vi "buildWaveform.vi"(8 "error in (no error)":errorcluster, 10 "Waveforms":T1, 11 "WaveformFactory in":refnum<class "WaveformFactory.lvclass">) -> (0 "error out":errorcluster, 2 "Waveform":refnum<class "IWaveform.lvclass">, 3 "WaveformFactory out":refnum<class "WaveformFactory.lvclass">)   [LabVIEW 2015, in "WaveformFactory.lvclass"]
uses:
  WaveformFactory.lvclass
  Typedefs/Waveform.ctl
  Waveforms/IWaveforms/IWaveform.lvclass
  WaveformFactory.lvclass/WaveformFactory.ctl
  Waveforms/PeriodicWave/PeriodicWave.lvclass
  Waveforms/ChirpWave/ChirpWave.lvclass
  Waveforms/GuassianNoiseWave/GuassianNoiseWave.lvclass
  Waveforms/TrapezoidalWave/TrapezoidalWave.lvclass
  Typedefs/FAMTTypedefs.lvlib
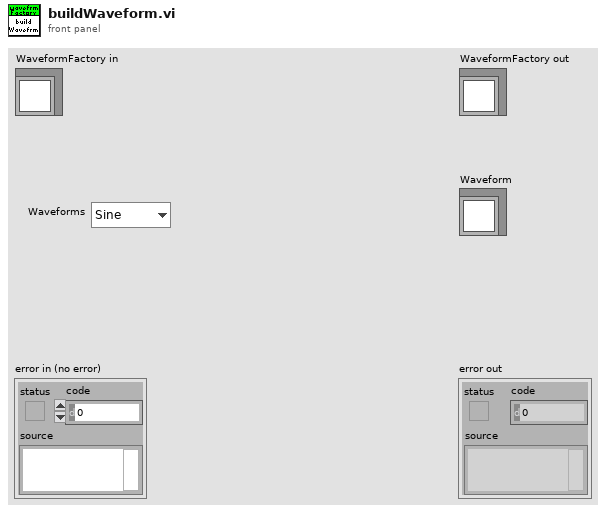
[diagram p1: front panel]
types:
  T1 = typedef "FAMTTypedefs.lvlib/Waveform.ctl" = enum16{"Sine", "Triangle", "Square", "Sawtooth", "Chirp", "Gaussian", "Trapezoid"}
  T2 = typedef "FAMTTypedefs.lvlib/Scan Settings.ctl" = cluster{"Amplitude Scan Settings":T3, "Rate Scan Settings":T4[], "Sample Count":u32, "Iterations":dbl, "Amplitude":dbl, "Offset":dbl, "Frequency":dbl[unit], "Waveform":T1, "F1":dbl[unit], "F2":dbl[unit], "Duty Cycle":dbl, "ILC Rate":dbl[unit], "Operator":string, "Scan Name":string, "Notes":string, "Ramp Time":dbl[unit], "Hold Time":dbl[unit], "Settling Time":dbl[unit], "Control Mode":T5, "FCV Rate":dbl}
  T3 = typedef "FAMTTypedefs.lvlib/Test Values.ctl" = cluster{"Start Value":dbl, "Stop Value":dbl, "Steps":u16}
  T4 = typedef "ILCCommon.lvlib/ILCConfiguration.lvlib/Scan Rates.ctl" = enum16{"50", "60", "100", "120", "200", "240", "300", "400", "480", "600", "1200", "2400", "4800"}
  T5 = typedef "FAMTTypedefs.lvlib/ControlMode.ctl" = enum16{"PSV", "FCV", "Both"}
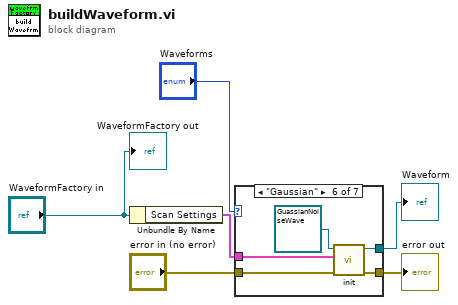
[diagram p0: block diagram]
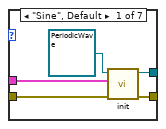
[diagram p2: hidden frame]
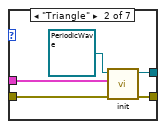
[diagram p3: hidden frame]
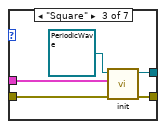
[diagram p4: hidden frame]
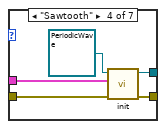
[diagram p5: hidden frame]
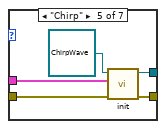
[diagram p6: hidden frame]
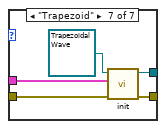
[diagram p7: hidden frame]
diagram:
  n1 = Unbundle By Name("WaveformFactory in") -> ("Scan Settings"=w3:T2)
  n2 = case shown="\"Gaussian\"" "Waveforms" {
    tunnel: w3 -> [w11 w16 w21 w26 w31 w32 w41]
    tunnel: [w7 w12 w17 w22 w27 w33 w37] -> w2
    tunnel: "error in (no error)" -> [w8 w13 w18 w23 w30 w35 w40]
    tunnel: [w9 w14 w19 w24 w28 w34 w39] -> w1
    frame "Sine", Default {
      n3 = call "init.vi"("error in (no error)"=w8, "Scan Settings"=w11, "PeriodicWave in"=refnum<class "PeriodicWave.lvclass"> refnum ("WaveformGenerator.lvclass")) -> ("error out"=w7:errorcluster, "PeriodicWave out"=w9:refnum<class "PeriodicWave.lvclass">)  [unwired: 7 in]
    }
    frame "Triangle" {
      n4 = call "init.vi"("error in (no error)"=w13, "Scan Settings"=w16, "PeriodicWave in"=refnum<class "PeriodicWave.lvclass"> refnum ("WaveformGenerator.lvclass")) -> ("error out"=w12:errorcluster, "PeriodicWave out"=w14:refnum<class "PeriodicWave.lvclass">)  [unwired: 7 in]
    }
    frame "Square" {
      n5 = call "init.vi"("error in (no error)"=w18, "Scan Settings"=w21, "PeriodicWave in"=refnum<class "PeriodicWave.lvclass"> refnum ("WaveformGenerator.lvclass")) -> ("error out"=w17:errorcluster, "PeriodicWave out"=w19:refnum<class "PeriodicWave.lvclass">)  [unwired: 7 in]
    }
    frame "Sawtooth" {
      n6 = call "init.vi"("error in (no error)"=w23, "Scan Settings"=w26, "PeriodicWave in"=refnum<class "PeriodicWave.lvclass"> refnum ("WaveformGenerator.lvclass")) -> ("error out"=w22:errorcluster, "PeriodicWave out"=w24:refnum<class "PeriodicWave.lvclass">)  [unwired: 7 in]
    }
    frame "Chirp" {
      n7 = call "init.vi"("error in (no error)"=w30, "Scan Settings"=w31, "ChirpWave in"=refnum<class "ChirpWave.lvclass"> refnum) -> ("error out"=w27:errorcluster, "ChirpWave out"=w28:refnum<class "ChirpWave.lvclass">)  [unwired: 7 in]
    }
    frame "Gaussian" {
      n8 = call "init.vi"("error in (no error)"=w35, "Scan Settings"=w32, "GuassianNoiseWave in"=refnum<class "GuassianNoiseWave.lvclass"> refnum) -> ("error out"=w33:errorcluster, "GuassianNoiseWave out"=w34:refnum<class "GuassianNoiseWave.lvclass">)  [unwired: 7 in]
    }
    frame "Trapezoid" {
      n9 = call "init.vi"("error in (no error)"=w40, "Scan Settings"=w41, "TrapezoidalWave in"=refnum<class "TrapezoidalWave.lvclass"> refnum) -> ("error out"=w37:errorcluster, "TrapezoidalWave out"=w39:refnum<class "TrapezoidalWave.lvclass">)  [unwired: 7 in]
    }
  }
  "error out" <- w2
  "Waveform" <- w1
  "WaveformFactory out" <- "WaveformFactory in"
